vi "onDestroy.vi"(8 "error in (no error)":errorcluster, 11 "Client in":refnum<class "Client.lvclass">) -> (0 "error out":errorcluster, 3 "Client out":refnum<class "Client.lvclass">)   [LabVIEW 2013, in "MQTT Server.lvlib" / "Client.lvclass"]
uses:
  Client.lvclass
  MQTT_Base/MQTT_Base.lvclass
  Client.lvclass/Client.ctl
  Server/Session/Session.lvclass
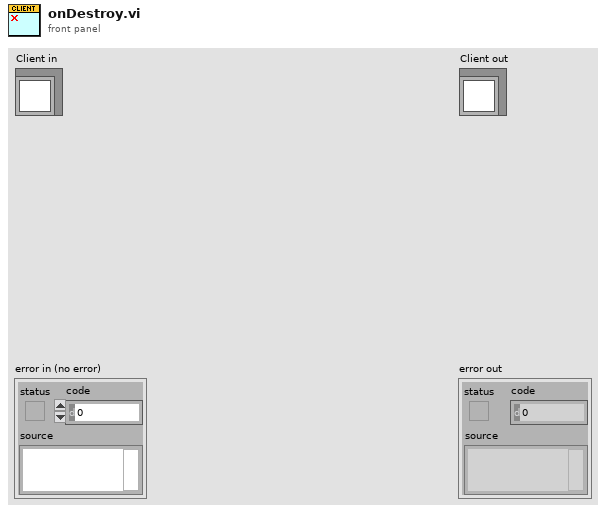
[diagram p1: front panel]
types:
  T1 = typedef "MQTT Server.lvlib/Client.lvclass/Public Events -- cluster.ctl" = cluster{"Connection Status":refnum<user-event>, "Connected":refnum<user-event>, "Application Message":refnum<user-event>}
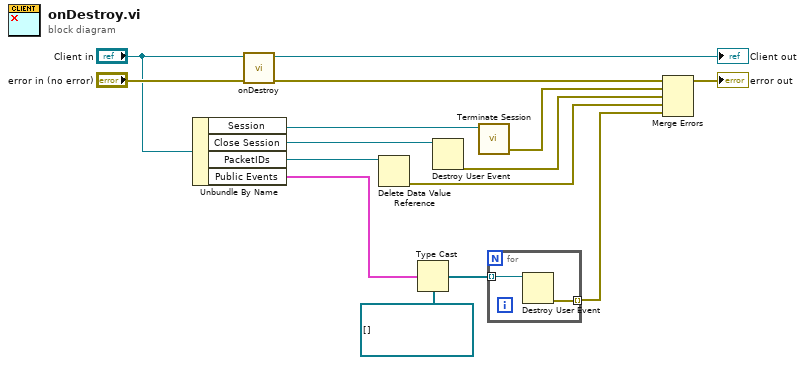
[diagram p0: block diagram]
diagram:
  n1 = Unbundle By Name("Client in") -> ("Session"=w11:refnum<class "Session.lvclass">, "Close Session"=w7:refnum<user-event>, "PacketIDs"=w12:refnum<data-value>, "Public Events"=w2:T1)
  n2 = call-parent "onDestroy.vi"("error in (no error)"="error in (no error)", "MQTT_Base in"="Client in") -> ("error out"=w10:errorcluster, "MQTT_Base out"=→"Client out":refnum<class "Client.lvclass">)  [unwired: 8 in]
  n3 = Delete Data Value Reference(data value reference=w12) -> (error out=w1:errorcluster)  [unwired: 1 in, 1 out]
  n4 = Type Cast(type=refnum<user-event>[] [], x=w2) -> (*(type *) &x=w5:refnum<user-event>[])
  n5 = Destroy User Event(user event=w7) -> (error out=w4:errorcluster)  [unwired: 1 in]
  n6 = call "Terminate Session.vi"("Session in"=w11) -> ("error out"=w8:errorcluster)  [unwired: 8 in, 2 out]
  n7 = for {
    tunnel: w5 -> [w17] mode=indexing
    tunnel: [w16] -> w3 mode=indexing
    n8 = Destroy User Event(user event=w17) -> (error out=w16:errorcluster)  [unwired: 1 in]
  }
  n9 = Merge Errors(w10, w8, w4, w1, w3) -> (→"error out":errorcluster)
